vi "test_average-z-data.vi"() -> ()   [LabVIEW 2015]
panel:
  out "mean is valid":bool
  out "MEAN":sgl
  out "Array":sgl[](array[numeric])
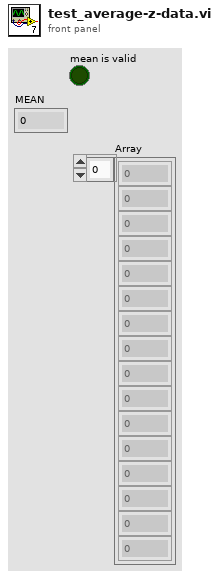
[diagram p1: front panel]
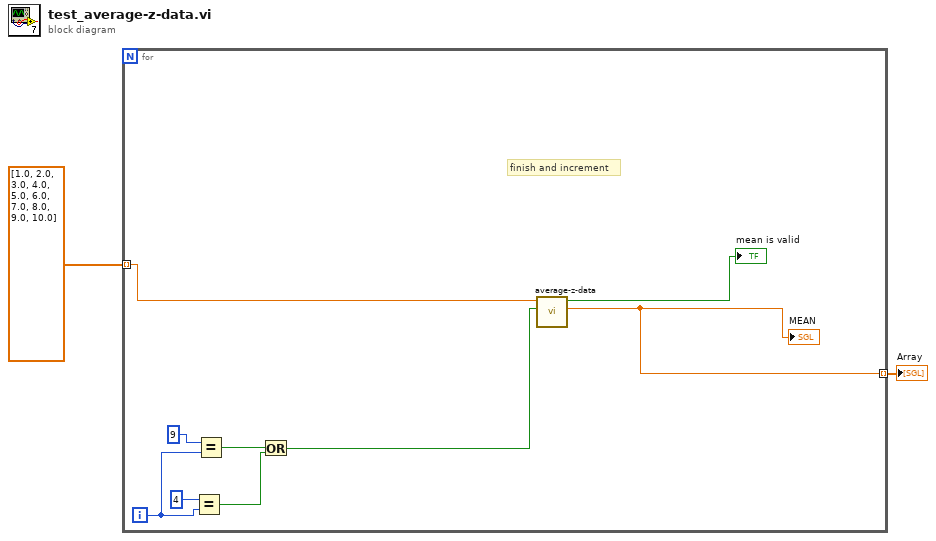
[diagram p0: block diagram]
diagram:
  n1 = for {
    tunnel: sgl[] [1.0, 2.0, 3.0, 4.0, 5.0, 6.0, 7.0, 8.0, 9.0, 10.0] -> [w5] mode=indexing
    tunnel: [w3] -> w1 mode=indexing
    i -> [w9]
    # "finish and increment"
    n2 = Equal?(x=4, y=w9) -> (x = y?=w6:bool)
    n3 = Equal?(x=9, y=w9) -> (x = y?=w8:bool)
    n4 = Or(x=w8, y=w6) -> (x .or. y?=w7:bool)
    n5 = call "average-z-data.vi"("Boolean"=w7, "z-data"=w5) -> ("MEAN"=w3:sgl, "mean is valid"=→"mean is valid":bool)  [unwired: 8 in]
    "MEAN" <- w3
  }
  "Array" <- w1
